vi "Test_FGV2.vi"() -> ()   [LabVIEW 2017]
panel:
  out "output":dbl
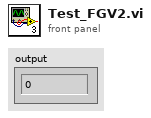
[diagram p1: front panel]
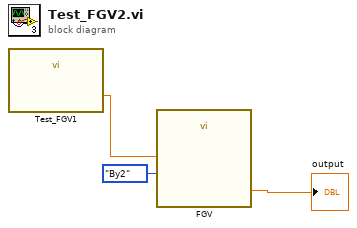
[diagram p0: block diagram]
diagram:
  n1 = call "Test_FGV1.vi"() -> ("output"=w3:dbl)  [unwired: 11 in]
  n2 = call "FGV.vi"("input"=w3, "mode"=enum16{"By1", "By2"}."By2") -> ("output"=→"output":dbl)  [unwired: 9 in]
